vi "Initialize.vi"(0 "VISA resource name":refnum<visa-resource-name>, 5 "ID Query (True)":bool=TRUE, 7 "Serial Configuration":T1={"Baud Rate (19200)"=19200, "Parity (0: None)"=0, "Data Bits (8)"=8, "Stop Bits (2.0)"=10} {"Stop Bits (2.0)" items=["1.0"=10, "2.0"=20]; "Data Bits (8)" items=["7"=7, "8"=8]; "Parity (0: None)" items=["None", "Odd", "Even"]; "Baud Rate (19200)" items=["4800"=4800, "9600"=9600, "19200"=19200, "57600"=57600, "115200"=115200]}, 9 "Reset (True)":bool=TRUE, 11 "error in (no error)":errorcluster) -> (4 "VISA resource name out":refnum<visa-resource-name>, 6 "Modulation Available":u32, 10 "Memory Available":u32, 15 "error out":errorcluster)   [LabVIEW 2020, in "MagnaDC.lvlib"]
doc: "Establishes communication with the instrument and optionally performs an instrument identification query and/or an instrument reset. It also places the instrument in a default state needed for other instrument driver operations. Therefore, call this VI before calling other instrument driver VIs for this instrument. Generally, you need to call the <b>Initialize</b> VI only once at the beginning of an application."
uses:
  MagnaDC.lvlib
panel:
  # "(c) 2004-2018 Magna-Power Electronics Inc.  ALL RIGHTS RESERVED."
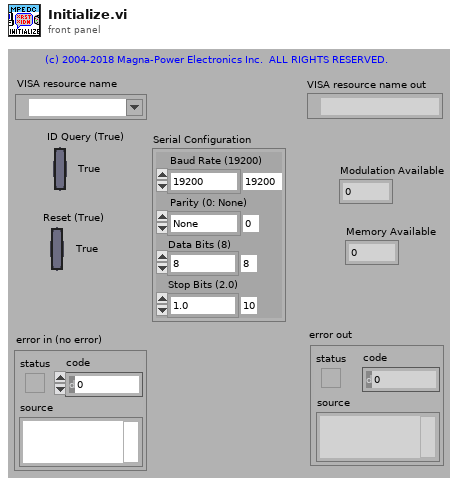
[diagram p1: front panel]
types:
  T1 = cluster{"Baud Rate (19200)":u32, "Parity (0: None)":u16, "Data Bits (8)":u16, "Stop Bits (2.0)":u16}
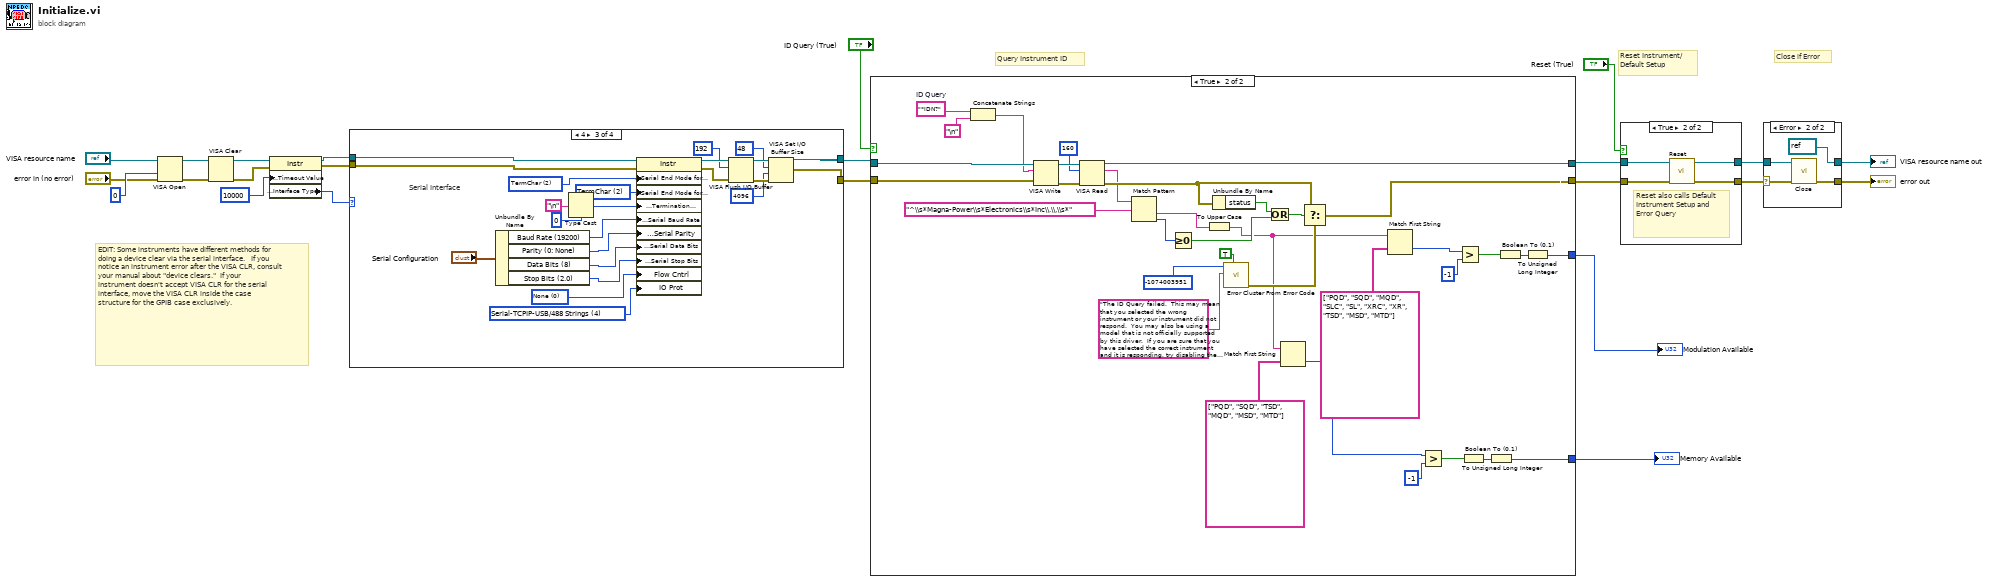
[diagram p0: block diagram]
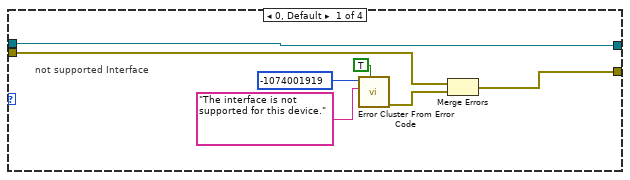
[diagram p2: hidden frame]
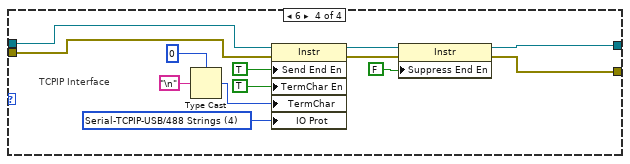
[diagram p4: hidden frame]
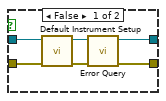
[diagram p6: hidden frame]
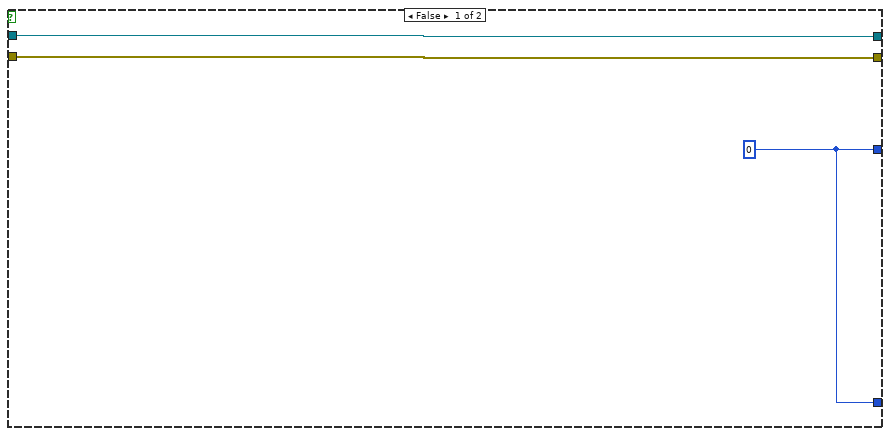
[diagram p7: hidden frame]
diagram:
  # "EDIT: Some instruments have different methods for doing a device clear via the serial interface.   If you notice an instrument error after the VISA CLR, consult your manual about \"device clears.\"  If your instrument doesn't accept VISA CLR for the serial interface, move the VISA CLR inside the case  structure for the GPIB case exclusively."
  # "Close if Error"
  # "Query Instrument ID"
  # "Reset Instrument/\nDefault Setup"
  n1 = VISA Open(access mode=u32 0, error in (no error)="error in (no error)", VISA resource name="VISA resource name") -> (VISA resource name=w13:refnum<visa-resource-name>, error out=w12:errorcluster)  [unwired: 2 in]
  n2 = VISA Clear(VISA resource name=w13, error in (no error)=w12) -> (VISA resource name out=w11:refnum<visa-resource-name>, error out=w10:errorcluster)
  n3 = property class="Instr"(reference=w11, error in=w10, "General Settings:Timeout Value"=u32 10000) -> (reference out=w8:refnum<visa-resource-name>, error out=w9:errorcluster, "Interface Information:Interface Type"=w7:u16)
  n4 = case shown="4" w7 {
    tunnel: [w30 w32 w52 w59] -> w6
    tunnel: [w26 w31 w49 w58] -> w5
    tunnel: w8 -> [w30 w32 w54 w68]
    tunnel: w9 -> [w25 w31 w55 w67]
    frame 0, Default {
      # "not supported Interface"
      n5 = call <vilib>:"Error Cluster From Error Code.vi"("show call chain? (False)"=TRUE, "error message (\"\")"="The interface is not supported for this device." ("Source (VI Name)"), "error code (0)"=-1074001919 ("Code")) -> ("error out"=w24:errorcluster)  [unwired: 6 in]
      n6 = Merge Errors(w25, w24) -> (w26:errorcluster)
    }
    frame 1 {
      # "GPIB Interface"
    }
    frame 4 {
      w38 = u16 0 items=["None", "XON/XOFF", "RTS/CTS", "XON/XOFF & RTS/CTS", "DTR/DSR", "XON/XOFF & DTR/DSR"] ("Serial Settings:Serial Flow Control")
      w39 = u16 4 items=["Normal"=1, "VXI/FDC"=2, "GPIB/HS488"=3, "Serial-TCPIP-USB/488 Strings"=4, "USBTMC/Vendor-Specific"=5] ("Message Based Settings:IO Protocol")
      w40 = u16 2 items=["None", "Last Bit", "TermChar", "Break"] ("Serial Settings:End Mode for Writes")
      w42 = u16 2 items=["None", "LastBit", "TermChar"] ("Serial Settings:Serial End Mode for Reads")
      # "Serial Interface"
      n7 = Unbundle By Name("Serial Configuration") -> ("Baud Rate (19200)"=w37:u32, "Parity (0: None)"=w36:u16, "Data Bits (8)"=w35:u16, "Stop Bits (2.0)"=w34:u16)
      n8 = Type Cast(type=u8 0, x="\n" ("Line Feed Constant")) -> (*(type *) &x=w41:u8)
      n9 = property class="Instr"(reference=w54, error in=w55, "Serial Settings:Serial End Mode for Reads"=w42, "Serial Settings:Serial End Mode for Writes"=w40, "Message Based Settings:Termination Character"=w41, "Serial Settings:Serial Baud Rate"=w37, "Serial Settings:Serial Parity"=w36, "Serial Settings:Serial Data Bits"=w35, "Serial Settings:Serial Stop Bits"=w34, "Flow Cntrl"=w38, "IO Prot"=w39) -> (reference out=w48:refnum<visa-resource-name>, error out=w51:errorcluster)
      n10 = VISA Flush I/O Buffer(VISA resource name=w48, mask (16)=u32 192, error in (no error)=w51) -> (VISA resource name out=w53:refnum<visa-resource-name>, error out=w50:errorcluster)
      n11 = VISA Set I/O Buffer Size(VISA resource name=w53, mask (16)=u32 48, size (4096)=u32 4096 ("size (0)"), error in (no error)=w50) -> (VISA resource name out=w52:refnum<visa-resource-name>, error out=w49:errorcluster)
    }
    frame 6 {
      w63 = u16 4 items=["Normal"=1, "VXI/FDC"=2, "GPIB/HS488"=3, "Serial-TCPIP-USB/488 Strings"=4, "USBTMC/Vendor-Specific"=5] ("Message Based Settings:IO Protocol")
      # "TCPIP Interface"
      n12 = Type Cast(type=u32 0, x="\n" ("Line Feed Constant")) -> (*(type *) &x=w64:u32)
      n13 = property class="Instr"(reference=w68, error in=w67, "Send End En"=TRUE ("Message Based Settings:Send End Enable"), "TermChar En"=TRUE ("Message Based Settings:Termination Character Enable"), "TermChar"=w64, "IO Prot"=w63) -> (reference out=w56:refnum<visa-resource-name>, error out=w57:errorcluster)
      n14 = property class="Instr"(reference=w56, error in=w57, "Suppress End En"=FALSE) -> (reference out=w59:refnum<visa-resource-name>, error out=w58:errorcluster)
    }
  }
  n15 = case shown="True" "ID Query (True)" {
    tunnel: [w70 w106] -> w22
    tunnel: [w71 w105] -> w23
    tunnel: w6 -> [w71 w95]
    tunnel: w5 -> [w70 w94]
    tunnel: [w69 w79] -> w2
    tunnel: [w69 w72] -> w1
    frame False {
      w69 = u32 0
    }
    frame True {
      w91 = "*IDN?"  # ID Query
      n16 = Concatenate Strings(w91, "\n") -> (w90:string)
      n17 = VISA Write(VISA resource name=w95, write buffer=w90, error in (no error)=w94) -> (VISA resource name out=w104:refnum<visa-resource-name>, error out=w103:errorcluster)  [unwired: 1 out]
      n18 = VISA Read(VISA resource name=w104, byte count=u32 160, error in (no error)=w103) -> (VISA resource name out=w105:refnum<visa-resource-name>, read buffer=w89:string, error out=w98:errorcluster)  [unwired: 1 out]
      n19 = Match Pattern(string=w89, regular expression="^\\s*Magna-Power\\s*Electronics\\s*Inc\\.\\,\\s*") -> (after substring=w85:string, offset past match=w87:i32)  [unwired: 1 in, 2 out]
      n20 = Greater Or Equal To 0?(x=w87) -> (x >= 0?=w86:bool)
      n21 = To Upper Case(1:w85) -> (0:w77:string)
      n22 = Unbundle By Name(w98) -> ("status"=w97:bool)
      n23 = call <vilib>:"Error Cluster From Error Code.vi"("show call chain? (False)"=TRUE, "error message (\"\")"="The ID Query failed.  This may mean that you selected the wrong instrument or your instrument did not respond.  You may also be using a model that is not officially supported by this driver.  If you are sure that you have selected the correct instrument and it is responding, try disabling the ID Query." ("Source (VI Name)"), "error code (0)"=-1074003951 ("Code")) -> ("error out"=w101:errorcluster)  [unwired: 6 in]
      n24 = Or(x=w97, y=w86) -> (x .or. y?=w96:bool)
      n25 = Match First String(2:string[] ["PQD", "SQD", "TSD", "MQD", "MSD", "MTD"] ("string array"), 3:w77) -> (0:w73:i32)  [unwired: 1 out]
      n26 = Select(t=w98, s=w96, f=w101) -> (s? t:f=w106:errorcluster)
      n27 = Match First String(2:string[] ["PQD", "SQD", "MQD", "SLC", "SL", "XRC", "XR", "TSD", "MSD", "MTD"] ("string array"), 3:w77) -> (0:w80:i32)  [unwired: 1 out]
      n28 = Greater?(x=w73, y=-1) -> (0:w75:bool)
      n29 = Greater?(x=w80, y=-1) -> (0:w82:bool)
      n30 = Boolean To (0,1)(Boolean=w75) -> (0, 1=w74:i16)
      n31 = To Unsigned Long Integer(number=w74) -> (unsigned 32bit integer=w72:u32)
      n32 = Boolean To (0,1)(Boolean=w82) -> (0, 1=w81:i16)
      n33 = To Unsigned Long Integer(number=w81) -> (unsigned 32bit integer=w79:u32)
    }
  }
  "Modulation Available" <- w2
  "Memory Available" <- w1
  n34 = case shown="True" "Reset (True)" {
    tunnel: w22 -> [w111 w115]
    tunnel: [w108 w114] -> w17
    tunnel: w23 -> [w112 w116]
    tunnel: [w109 w113] -> w18
    frame False {
      n35 = call "Default Instrument Setup.vi"("error in (no error)"=w111, "VISA resource name"=w112) -> ("error out"=w107:errorcluster, "VISA resource name out"=w110:refnum<visa-resource-name>)  [unwired: 8 in]
      n36 = call "Error Query.vi"("error in (no error)"=w107, "VISA resource name"=w110) -> ("error out"=w108:errorcluster, "VISA resource name out"=w109:refnum<visa-resource-name>)  [unwired: 6 in, 2 out]
    }
    frame True {
      # "Reset also calls Default Instrument Setup and Error Query"
      n37 = call "Reset.vi"("error in (no error)"=w115, "VISA resource name"=w116) -> ("error out"=w114:errorcluster, "VISA resource name out"=w113:refnum<visa-resource-name>)  [unwired: 8 in]
    }
  }
  n38 = case shown="Error" w17 {
    selector: w17 -> [w117 w120]
    tunnel: w18 -> [w118 w121]
    tunnel: [w118 refnum<visa-resource-name> refnum ("VISA resource name out")] -> w20
    tunnel: [w117 w122] -> w19
    frame No Error {
    }
    frame Error {
      n39 = call "Close.vi"("error in (no error)"=w120, "VISA resource name"=w121) -> ("error out"=w122:errorcluster)  [unwired: 9 in]
    }
  }
  "VISA resource name out" <- w20
  "error out" <- w19
